vi "number5-sub3.vi"(4 "Numeric":i32, 6 "Array":i32[](array[numeric])) -> (3 "Array 2":i32[][](array[numeric]))   [LabVIEW 2014]
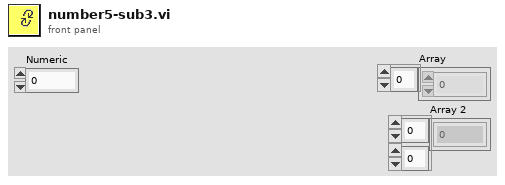
[diagram p1: front panel]
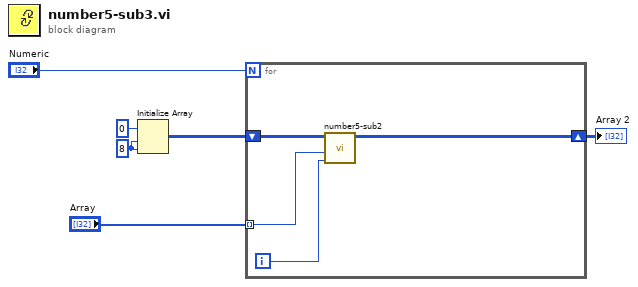
[diagram p0: block diagram]
diagram:
  w5 = 8 ("dimension size")
  n1 = Initialize Array(0 ("element"), w5, w5) -> (w3:i32[][])
  n2 = for {
    N: "Numeric" -> [_]
    shift-right: [w7] -> w1
    shift-left: w3 -> [w10]
    tunnel: "Array" -> [w9] mode=indexing
    i -> [w8]
    n3 = call "number5-sub2.vi"("Numeric"=w8, "Numeric 2"=w9, "array"=w10) -> ("array 2"=w7:i32[][])  [unwired: 4 in]
  }
  "Array 2" <- w1
